vi "Undeploy Libraries.vi"(8 "Error In":errorcluster, 10 "SV-Library Paths":path[](array[path]), 11 "CS++DSCManager in":refnum<class "CS++DSCManager.lvclass">) -> (0 "Error Out":errorcluster, 3 "CS++DSCManager out":refnum<class "CS++DSCManager.lvclass">)   [LabVIEW 2016, in "CS++DSCManager.lvlib" / "CS++DSCManager.lvclass"]
doc: "Removes the variables defined in multiple LabVIEW project libraries from the Shared Variable Engine (SVE) on the host computer."
uses:
  CS++DSCManager.lvclass
  <vilib>/lvdsc/process/internal/PRC_UndeployLibraries.vi
  <vilib>/lvdsc/NI_DSC.lvlib
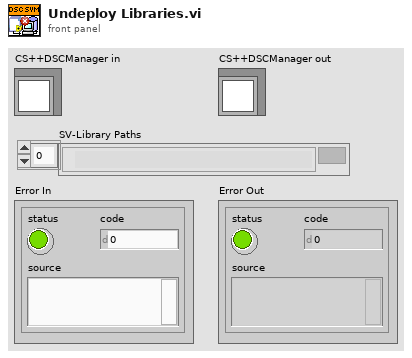
[diagram p1: front panel]
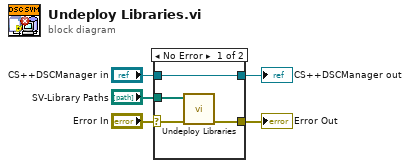
[diagram p0: block diagram]
diagram:
  n1 = case shown="No Error" "Error In" {
    selector: "Error In" -> [w9 w11]
    tunnel: [w6 w11] -> w4
    tunnel: [w7 w10] -> w2
    tunnel: "CS++DSCManager in" -> [w7 w10]
    tunnel: "SV-Library Paths" -> [w8 _]
    frame No Error {
      n2 = call-poly <vilib>:"Undeploy Libraries.vi"("error in (no error)"=w9, "library paths"=w8) -> ("error out"=w6:errorcluster)  [unwired: 7 in]
    }
    frame Error {
    }
  }
  "Error Out" <- w4
  "CS++DSCManager out" <- w2
